vi "overlay_generation.vi"(5 "center radius":dbl, 6 "Color":u32(colorbox)=16448250, 7 "number of rings":i32, 10 "Image Src":T1, 11 "fringe preview on":bool) -> ()   [LabVIEW 2011]
doc: "Creates Overlay pattern to help with the alignment of the setup. The input image is copied and a new memory space is create to hold the overlay image in order to keep the originally created pattern."
uses:
  <vilib>/vision/Image Controls.llb/IMAQ Image.ctl
  global_vars.vi
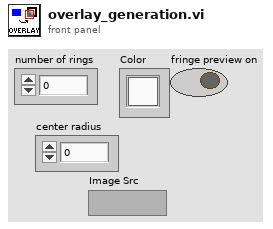
[diagram p1: front panel]
types:
  T1 = typedef "IMAQ Image.ctl" = refnum<image>
  T2 = cluster{"Desired Font (Application)":enum16{"User-specified Font", "Application Font", "System Font", "Dialog Font"}, "[User-specified Font]":cluster{"Font Name":string, "Size":i16, "Strikeout?":bool, "Italic?":bool, "Underline?":bool, "Outline?":bool, "Shadow?":bool, "Bold?":bool, "Rotation Angle":dbl}, "Horizontal Alignment":i16, "Vertical Alignment":i16}
  T3 = cluster{"Numeric Control":dbl, "Numeric Control":dbl, "Numeric Control":dbl, "Numeric Control":dbl}
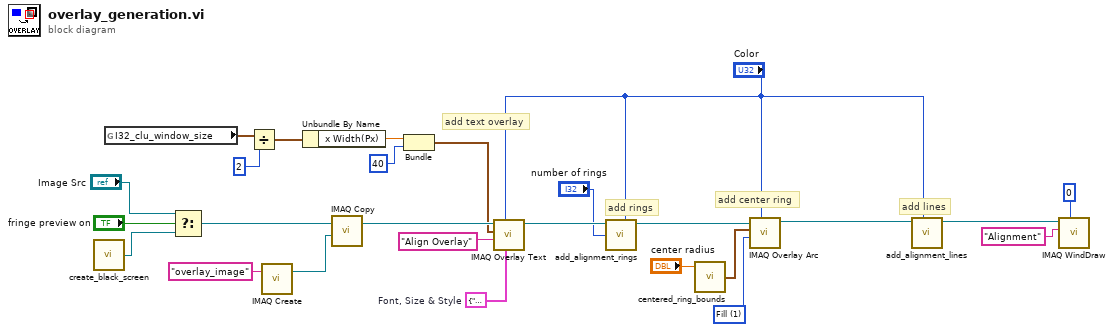
[diagram p0: block diagram]
diagram:
  w9 = u32 1 items=["Frame", "Fill"] ("Drawing Mode (Frame)")
  w25 = T2 {"Desired Font (Application)"=enum."User-specified Font", "[User-specified Font]"={"Font Name"="Arial", "Size"=30, "Strikeout?"=FALSE, "Italic?"=FALSE, "Underline?"=FALSE, "Outline?"=FALSE, "Shadow?"=FALSE, "Bold?"=TRUE, "Rotation Angle"=0.0}, "Horizontal Alignment"=1, "Vertical Alignment"=2}  # Font, Size & Style
  # "add lines"
  # "add center ring"
  # "add rings"
  # "add text overlay"
  n1 = call "create_black_screen.vi"() -> ("img_black_screen"=w6:T1)  [unwired: 5 in]
  n2 = global read "global_vars.vi" "I32_clu_window_size"() -> (w18:cluster{"x Width(Px)":i32, "y height(Px)":i32})
  n3 = Select(t="Image Src", s="fringe preview on", f=w6) -> (s? t:f=w5:T1)
  n4 = Divide(x=w18, y=2 ("y height(Px)")) -> (x/y=w17:cluster{"x Width(Px)":dbl, "y height(Px)":dbl})
  n5 = call "IMAQ Create"("Image Name"="overlay_image") -> ("New Image"=w22:T1)  [unwired: 4 in, 1 out]
  n6 = Unbundle By Name(w17) -> ("x Width(Px)"=w16:dbl)
  n7 = call "IMAQ Copy"("Image Dst"=w22, "Image Src"=w5) -> ("Image Dst Out"=w23:T1)  [unwired: 4 in, 1 out]
  n8 = Bundle("x Width(Px)"=w16, 40) -> (w21:cluster{"x Width(Px)":dbl, i32})  [unwired: 1 in]
  n9 = call "IMAQ Overlay Text"("Text Color (black)"="Color", "Font, Size & Style"=w25, "String"="Align Overlay", "Origin"=w21, "Image"=w23) -> ("Image Out"=w15:T1)  [unwired: 5 in, 1 out]
  n10 = call "add_alignment_rings.vi"("Color"="Color", "number of rings"="number of rings", "Image in"=w15) -> ("Image Out"=w11:T1)  [unwired: 6 in]
  n11 = call "centered_ring_bounds.vi"("radius R"="center radius") -> ("Bounding Rectangle"=w13:T3)  [unwired: 4 in]
  n12 = call "IMAQ Overlay Arc"("Color"="Color", "Drawing Mode (Frame)"=w9, "Bounding Rectangle"=w13, "Image"=w11) -> ("Image Out"=w10:T1)  [unwired: 6 in, 1 out]
  n13 = call "add_alignment_lines.vi"("Color"="Color", "Image in"=w10) -> ("Image out"=w1:T1)  [unwired: 9 in]
  n14 = call "IMAQ WindDraw"("Window Number (0...15)"=0, "Title"="Alignment", "Image"=w1) -> ()  [unwired: 7 in, 2 out]
